vi "Error Channels Write Array.vi"(8 "error in (no error)":errorcluster, 10 "Error Channels STS":i32, 11 "Error Channels in":refnum<class "Error Channels.lvclass">) -> (0 "error out":errorcluster, 3 "Error Channels out":refnum<class "Error Channels.lvclass">)   [LabVIEW 2023, in "Error Channels.lvclass"]
uses:
  Error Channels.lvclass
  Error Channels.lvclass/Error Channels.ctl
  <vilib>/ADAS Replay HIL/Channels/Tag Wrapper/Polymorphic/Write Channel (I32).vi
  <vilib>/ADAS Replay HIL/Channels/Tag Wrapper/Polymorphic/Write Channel (I32).vi/cccb8e89-591f-4bb4-9d4e-ae06ba1f5498.vi
  <vilib>/ADAS Replay HIL/Channels/Tag Wrapper/Polymorphic/Write Channel (I32).vi/cccb8e89-591f-4bb4-9d4e-ae06ba1f5498.vi/4bc1c15b-36ab-481f-b8dd-c64075ce723a.vi
  <vilib>/ADAS Replay HIL/Channels/Tag Wrapper/Polymorphic/Write Channel (I32).vi/cccb8e89-591f-4bb4-9d4e-ae06ba1f5498.vi/d83cb72b-7713-41fc-a3d1-682de79cf574.vi
  <vilib>/ADAS Replay HIL/Channels/Tag Wrapper/Tag Wrapper.lvlib
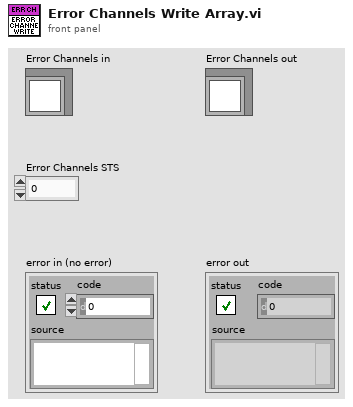
[diagram p1: front panel]
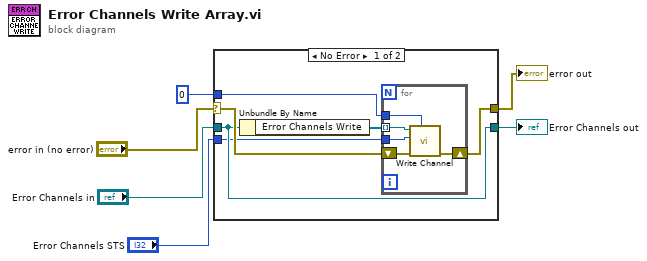
[diagram p0: block diagram]
diagram:
  n1 = case shown="No Error" "error in (no error)" {
    selector: "error in (no error)" -> [w12 w19]
    tunnel: [w11 w19] -> w4
    tunnel: [w10 w18] -> w5
    tunnel: "Error Channels in" -> [w10 w18]
    tunnel: "Error Channels STS" -> [w8 _]
    tunnel: 0 ("Timeout (ms)") -> [w7 _]
    frame No Error {
      n2 = Unbundle By Name(w10) -> ("Error Channels Write"=w9:refnum<k21>[])
      n3 = for {
        shift-right: [w16] -> w11
        shift-left: w12 -> [w17]
        tunnel: w9 -> [w15] mode=indexing
        tunnel: w8 -> [w14]
        tunnel: w7 -> [w13]
        n4 = call-poly <vilib>:"Write Channel.vi"("Timeout (ms)"=w13, "error in"=w17, "Value to Write"=w14, "ADAS HIL Channel in"=w15) -> ("error out"=w16:errorcluster)  [unwired: 5 in, 2 out]
      }
    }
    frame Error {
    }
  }
  "error out" <- w4
  "Error Channels out" <- w5
